vi "MD5 Message Digest__ogtk.vi"   [LabVIEW 2016]
doc: "Implements the MD5 algorithm to produce a 128-Bit Hash condensed representation of a message or a data file.\n\nPolymorphic VI can output MD5 Hash as Binary String or Hexadeximal String."
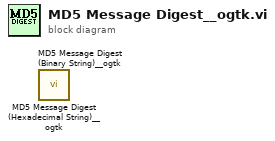
[diagram p0: block diagram]
diagram:
  n1 = call <userlib>:"MD5 Message Digest (Hexadecimal String)__ogtk.vi"() -> ()  [unwired: 1 in, 1 out]
  n2 = call <userlib>:"MD5 Message Digest (Binary String)__ogtk.vi"() -> ()  [unwired: 1 in, 1 out]
